vi "Preview_Build.vi"(8 "error in (no error)":errorcluster, 11 "Build in":refnum<class "AB_EXE.lvclass">) -> (0 "error out":errorcluster, 1 "GeneratedFiles":path[](array[path]), 3 "Build out":refnum<class "AB_EXE.lvclass">, 4 "GeneratedFileGUIDs":string[](array[string]), 5 "OutputDirectory":path)   [LabVIEW 2020, in "AB_EXE.lvclass"]
uses:
  <vilib>/AppBuilder/AB_Classes/EXE/AB_EXE.lvclass
  e:/builds/penguin/labview/branches/2020/dev/dist/vi.lib/AppBuilder/AB_Classes/Build/AB_Build.lvclass
  <vilib>/AppBuilder/AB_Classes/EXE/AB_EXE.lvclass/AB_EXE.ctl
  <vilib>/AppBuilder/AB_Classes/Application/AB_Application.lvclass
  <vilib>/AppBuilder/AB_Classes/Build/AB_Build.lvclass
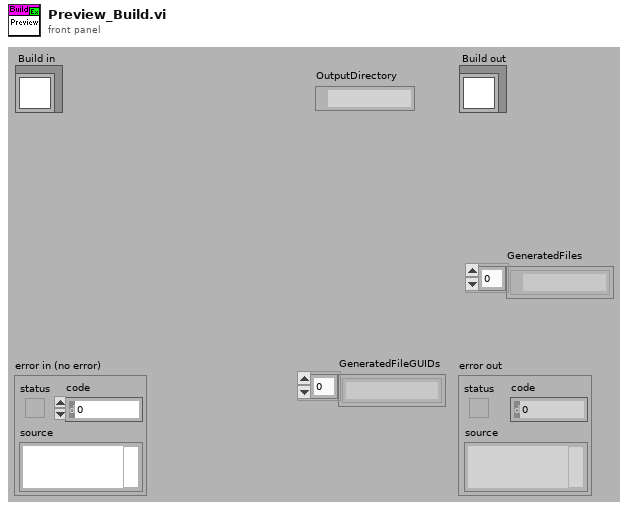
[diagram p1: front panel]
types:
  T1 = enum32{"invalid OS target", "Mac OS", "Windows 3.1", "Windows 95/NT", "Solaris 1", "Solaris 2", "HP-UX", "PowerMAX", "Linux", "Irix", "Rhapsody", "BeOS", "AIX", "OSF1", "VxWorks", "PharLap", "Carbon", "RTX", "Windows x64", "Linux x64", "Mac OS X x64"}
  T2 = typedef "AB_Build.ctl" = cluster{"buildSpecName":string, "buildSpecDescription":string, "destinations":refnum<class "AB_Destination.lvclass">[], "exclusionOption":T3, "defaultLanguage":string, "supportedLanguages":string[], "excludedDirectories":path[], "buildContext":refnum<vi>, "buildObject":T4, "preview":bool, "programatic":bool, "progressBarEvents":T5, "userLog_Path":path, "preActionID":string, "preAction_Path":path, "postActionID":string, "postAction_Path":path, "eng_checkForBrokenVIs?":bool, "eng_verboseLinkerErrors?":bool, "localDest_Path":path, "targetDest_Path":path, "removeVIObject":u16, "cache":refnum<class "PreviewCache.lvclass">, "use cache":bool, "previewCache_ID":string, "buildCache_ID":string, "eng_TempLocalDest_Path":path, "eng_collectDependencies?":bool, "versionInfo":cluster{"buildVersion":cluster{"major":u16, "minor":u16, "patch":u16, "build":u16}, "autoIncrement":bool}, "eng_enableVIChecksums":bool}
  T3 = typedef "AB_Exclusion_Option.ctl" = cluster{"typedefs":bool, "polymorphicVIs":bool, "unusedLibraryItems":bool, "modifyLibraryFile":bool, "edit-timeDependencies":bool, "inlineVIs":bool, "dependent PPLs":bool, "dependent DLLs":bool}
  T4 = typedef "ItemRef.ctl" = u64
  T5 = typedef "provcom_ProgressBar_Events.ctl" = cluster{"newJob":refnum<user-event>, "newItem":refnum<user-event>, "errorMsg":T6, "cancel":refnum<user-event>}
  T6 = typedef "mxLvBuildError.ctl" = refnum<user-event>
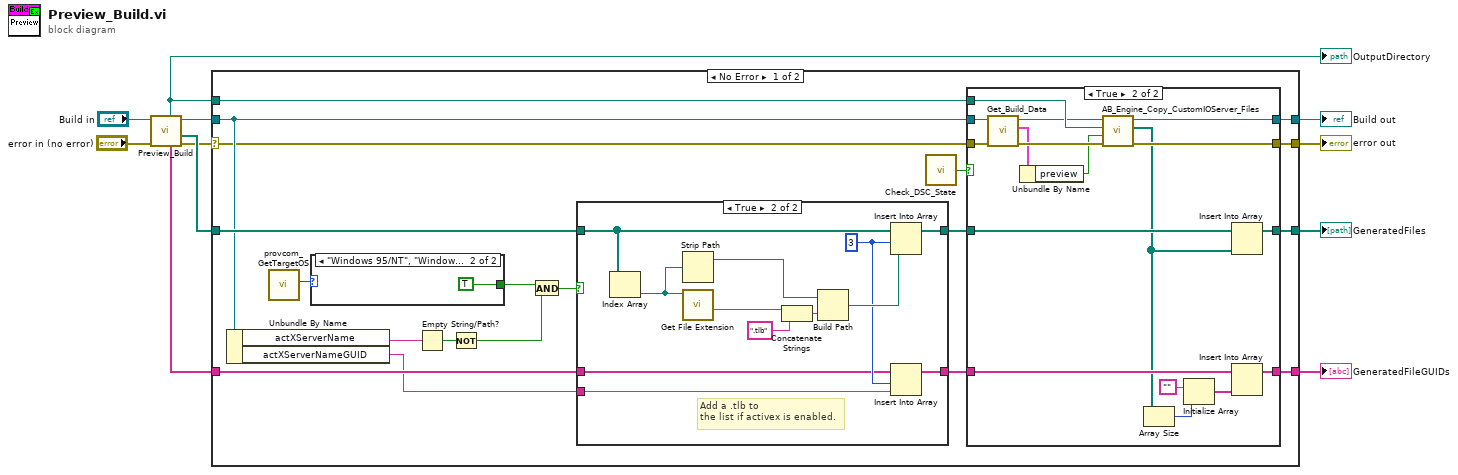
[diagram p0: block diagram]
diagram:
  n1 = call-parent "Preview_Build.vi"("error in (no error)"="error in (no error)", "Build in"="Build in") -> ("error out"=w4:errorcluster, "GeneratedFiles"=w9:path[], "Build out"=w5:refnum<class "AB_EXE.lvclass">, "GeneratedFileGUIDs"=w7:string[], "OutputDirectory"=w1:path)  [unwired: 5 out]
  "OutputDirectory" <- w1
  n2 = case shown="No Error" w4 {
    selector: w4 -> [w18 w69]
    tunnel: w9 -> [w27 w68]
    tunnel: [w14 w68] -> w8
    tunnel: w7 -> [w25 w67]
    tunnel: [w12 w67] -> w6
    tunnel: w5 -> [w20 w70]
    tunnel: [w17 w69] -> w3
    tunnel: [w19 w70] -> w2
    tunnel: w1 -> [w16 _]
    frame No Error {
      n3 = Unbundle By Name(w20) -> ("actXServerName"=w26:string, "actXServerNameGUID"=w24:string)
      n4 = call <resource>:"provcom_GetTargetOS.vi"() -> ("App.TargetOS"=w23:T1)  [unwired: 11 out]
      n5 = case shown="\"Windows 95/NT\", \"Windows x64\"" w23 {
        tunnel: [_ TRUE] -> w22
        frame Default {
        }
        frame "Windows 95/NT", "Windows x64" {
        }
      }
      n6 = Empty String/Path?(string/path=w26) -> (empty?=w29:bool)
      n7 = Not(x=w29) -> (.not. x?=w28:bool)
      n8 = And(x=w22, y=w28) -> (x .and. y?=w30:bool)
      n9 = case shown="True" w30 {
        tunnel: [w54 w62] -> w15
        tunnel: w27 -> [w54 w64]
        tunnel: w25 -> [w53 w60]
        tunnel: w24 -> [_ w59]
        tunnel: [w53 w58] -> w13
        frame False {
        }
        frame True {
          w61 = 3 ("index")
          # "Add a .tlb to\nthe list if activex is enabled."
          n10 = Index Array(array=w64) -> (element=w57:path)  [unwired: 1 in]
          n11 = Strip Path(path=w57) -> (stripped path=w56:path)  [unwired: 1 out]
          n12 = call <vilib>:"Get File Extension.vi"("file"=w57) -> ("filename without extension"=w55:string)  [unwired: 1 in, 9 out]
          n13 = Concatenate Strings(w55, ".tlb" ("string")) -> (w65:string)
          n14 = Build Path(base path=w56, name or relative path=w65) -> (appended path=w63:path)
          n15 = Insert Into Array(array=w64, index=w61, new element=w63) -> (w62:path[])
          n16 = Insert Into Array(array=w60, index=w61, new element=w59) -> (w58:string[])
        }
      }
      n17 = call <vilib>:"Check_DSC_State.vi"() -> ("active"=w21:bool)  [unwired: 1 out]
      n18 = case shown="True" w21 {
        tunnel: w20 -> [w34 w38]
        tunnel: w18 -> [w33 w40]
        tunnel: [w34 w51] -> w19
        tunnel: [w33 w50] -> w17
        tunnel: w16 -> [_ w49]
        tunnel: w15 -> [w32 w46]
        tunnel: w13 -> [w31 w44]
        tunnel: [w32 w45] -> w14
        tunnel: [w31 w43] -> w12
        frame False {
        }
        frame True {
          n19 = call <vilib>:"Get_Build_Data.vi"("error in (no error)"=w40, "Class in"=w38) -> ("error out"=w39:errorcluster, "data"=w36:T2, "Class out"=w37:refnum<class "AB_EXE.lvclass">)  [unwired: 7 out]
          n20 = Unbundle By Name(w36) -> ("preview"=w35:bool)
          n21 = call <vilib>:"AB_Engine_Copy_CustomIOServer_Files.vi"("error in (no error)"=w39, "Preview?"=w35, "OutputDirectory"=w49, "Build in"=w37) -> ("error out"=w50:errorcluster, "Dependent File Path Array"=w42:path[], "Build out"=w51:refnum<class "AB_EXE.lvclass">)  [unwired: 5 out]
          n22 = Array Size(array=w42) -> (size(s)=w48:i32)
          n23 = Initialize Array("", w48) -> (w41:string[])
          n24 = Insert Into Array(array=w46, new element=w42) -> (w45:path[])  [unwired: 1 in]
          n25 = Insert Into Array(array=w44, new element=w41) -> (w43:string[])  [unwired: 1 in]
        }
      }
    }
    frame Error {
    }
  }
  "error out" <- w3
  "GeneratedFiles" <- w8
  "Build out" <- w2
  "GeneratedFileGUIDs" <- w6
